vi "CompareWfm.vi"() -> ()   [LabVIEW 2022 SP3]
uses:
  <vilib>/Native 3D Graph/xcontrol/3DPC_SurfacePlot.xctl
  PreferencesControl.ctl
  <vilib>/Native 3D Graph/classes/Base Datatype.lvclass
panel:
  in  "Tab Control 2":enum32{"FRF", "Phase", "Nyquist"}(tab)
  out "Average FRF":cluster{dbl, "df":dbl, dbl[]}[](graph)
  out "Coherence":cluster{dbl, "df":dbl, dbl[]}(graph)
  in  "Remember":bool
  in  "Save":bool
  out "Phase":cluster{"t0":dbl, "dt":dbl, "Y":dbl[]}(graph)
  out "Energy":cluster{"x0":dbl, "df":dbl, dbl[]}[](graph)
  out "Nyquist Plot":cluster{dbl[], dbl[]}(graph)
  out "3D Nyquist":refnum<class "Base Datatype.lvclass">[](xcontrol)
  in  "Method":enum16{"Sqrt(H1H2)", "H1", "H2"}(ring)
  in  "sort by":enum16{"Title", "Hammer Hit"}(ring)
  in  "revert":bool
  in  "Tab Control":enum32{"Graphs", "Setttings", "Manipulation"}(tab)
  out "Mic Spectrum":cluster{dbl, "df":dbl, "FFT {X}":dbl[]}[](graph)
  out "Hammer Data":cluster{dbl, "dt":dbl, "Y":dbl[]}[](graph)
  out "Hammer Spectrum":cluster{dbl, "df":dbl, "FFT {X}":dbl[]}[](graph)
  out "Microphone Data":cluster{dbl, "dt":dbl, "Y":dbl[]}[](graph)
  in  "View":u16(ring) items=["Raw", "Volts", "Units (Pa, N, etc)"]
  in  "Settings":T1={"Name of test"="", "Date"=timestamp(0 s since 1904-01-01), "Location"="", "Template"="", "Soundcard"="", "resolution"=32, "Sampling rate"=48000, "Ch1 Gain "=25.0, "Ch2 Gain"=10.0, "Sample time (s)"=0.3, "Pre-trigger (s)"=0.01, "Hammer Threshold"=10.0, "Positions"=12, "Taps/Position"=5, "Set Names"="", "Freq resolution"=10.0, "Hammer cutoff"=0.0, "Mic cutoff"=0.0, "Double bounce "=0.0, "Hammer Cal"=10.0, "dB Offset"=0.0, "Accel Cal"=10.0, "Vibrometer Cal"=0.0, "Mic Cal"=0.0, "Output"=2, "Voltage Cal"=1.0, "Vibrometer Port"="ASRL27::INSTR", "Range"=4, "High Pass"=2, "Bandwidth"=4, "X Range"=[], "Y Range"=[], "dB Spread"=0.0, "Trigger"=0, "Ch_1"=25, "Ch_2"=25, "flip?"=FALSE, "60Hz"=FALSE, "Time offset"=0.0, "Piezo Cal"=1.0, "Default Notes"=""} {"Ch_2" min=1 step=1; "Ch_1" min=1 max=100 step=1; "Trigger" items=["Hammer (force)", "Self-tap", "Spacebar"]; "Bandwidth" items=["1 kHz"=1, "5 kHz"=5, "10 kHz"=10, "25 kHz"=25, "50 kHz"=50, "100 kHz"=100]; "High Pass" items=["Off", "13 Hz", "104 Hz"]; "Range" items=["10 mm/s"=1, "20 mm/s"=2, "50 mm/s"=5, "100 mm/s"=10, "200 mm/s"=20, "500 mm/s"=50, "1 m/s"=100, "2 m/s"=200]; "Output" items=["Accelerometer", "Speed (from acceleration)", "Microphone", "Vibrometer", "Piezo"]; "Voltage Cal" format="%#_13g"; "Ch2 Gain" format="%#_13g"; "Ch1 Gain" format="%#_13g"; "Double bounce" min=0.0; "Mic cutoff" min=0.0 format="%#_4g"; "Hammer cutoff" min=0.0 format="%#_4g"; "Freq resolution" min=0.0; "Pre-trigger (s)" format="%#_13g"; "Date" format="%<%H:%M\n%d/%m/%y>T"; "resolution" items=["16 bit"=16, "24 bit"=24, "32 bit"=32]; "Sampling rate" items=["22050 samp/s"=22050, "44100 samp/s"=44100, "48000 samp/s"=48000]}
  in  "Range":cluster{dbl, dbl}(slide)={0.0, 2.4242424242424243} scale=0.0..22000.0
  in  "Vibrometer delay (msec)":dbl(slide) scale=0.2..0.3
  in  "dB Spread":dbl=40.0
  out "Path To Raw Folder":path
  in  "Test Name":string(combo)
  in  "Instrument Name":string(combo)
  in  "Raw wfm Files":i32[](listbox)
  # "Hz"
  # "dB"
  # "dB"
  # "sec"
  # "sec"
  # "mV/Pa"
  # "mV/m/s2"
  # "mV/mm/s"
  # "V/N"
  # "sec"
  # "sec"
  # "mV/N"
  # "a.u."
  # "a.u."
  # "sec"
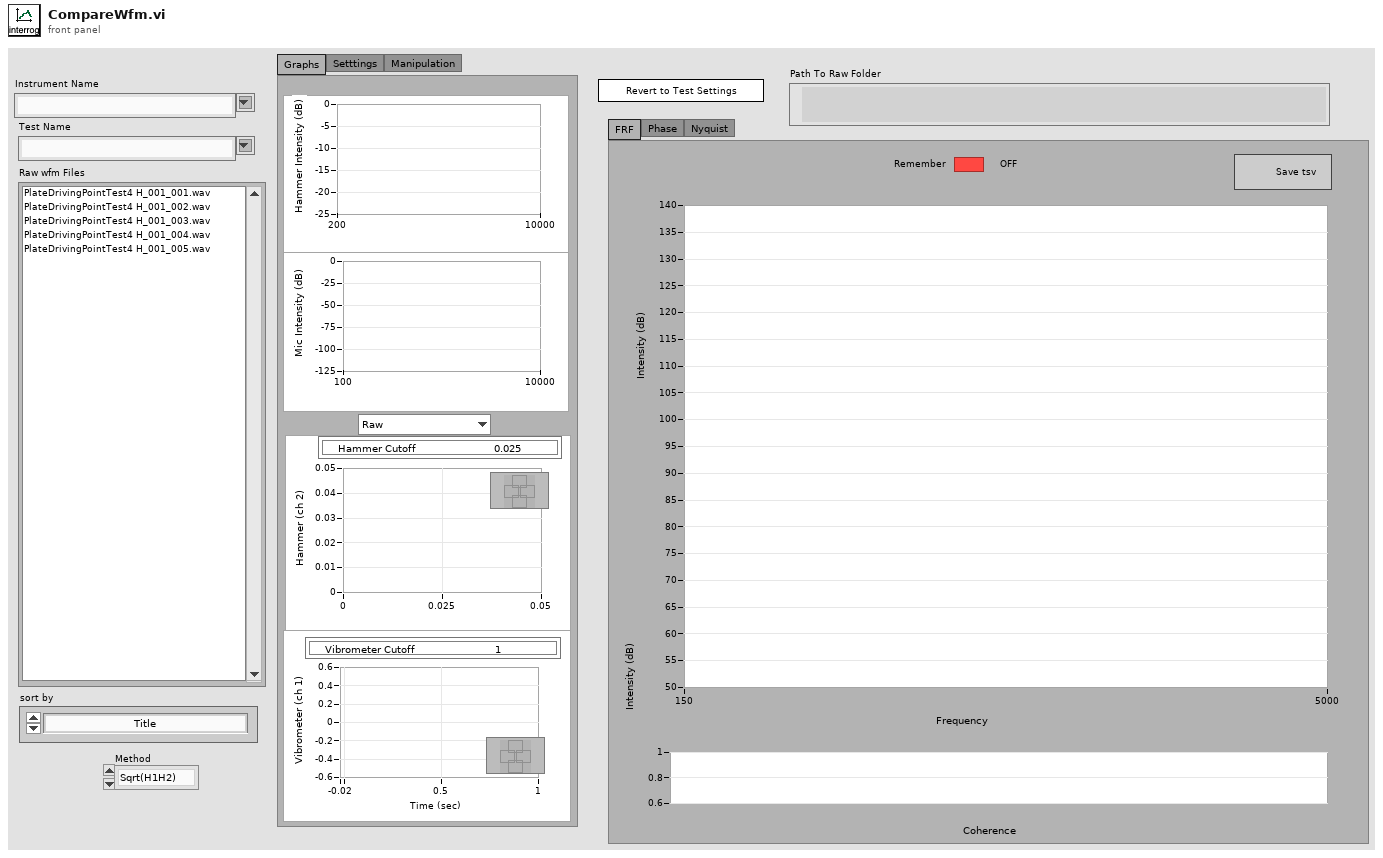
[diagram p1: front panel]
types:
  T1 = typedef "PreferencesControl.ctl" = cluster{"Name of test":string, "Date":timestamp, "Location":string, "Template":string, "Soundcard":string, "resolution":u16, "Sampling rate":u16, "Ch1 Gain ":dbl, "Ch2 Gain":dbl, "Sample time (s)":dbl, "Pre-trigger (s)":dbl, "Hammer Threshold":dbl, "Positions":i16, "Taps/Position":i16, "Set Names":string, "Freq resolution":dbl, "Hammer cutoff":dbl, "Mic cutoff":dbl, "Double bounce ":dbl, "Hammer Cal":dbl, "dB Offset":dbl, "Accel Cal":dbl, "Vibrometer Cal":dbl, "Mic Cal":dbl, "Output":u16, "Voltage Cal":dbl, "Vibrometer Port":refnum<visa-resource-name>, "Range":u16, "High Pass":u16, "Bandwidth":u16, "X Range":cluster{"Minimum":dbl, "Maximum":dbl, "Increment":dbl, "Minor Increment":dbl, "Start":dbl}[], "Y Range":cluster{"Minimum":dbl, "Maximum":dbl, "Increment":dbl, "Minor Increment":dbl, "Start":dbl}[], "dB Spread":dbl, "Trigger":u16, "Ch_1":u8, "Ch_2":u8, "flip?":bool, "60Hz":bool, "Time offset":dbl, "Piezo Cal":dbl, "Default Notes":string}
  T2 = typedef "LVRangeTypeDef.ctl" = cluster{"Minimum":dbl, "Maximum":dbl, "Increment":dbl, "Minor Increment":dbl, "Start":dbl}
  T3 = enum8{"Enabled", "Disabled", "Disabled and Grayed Out"}
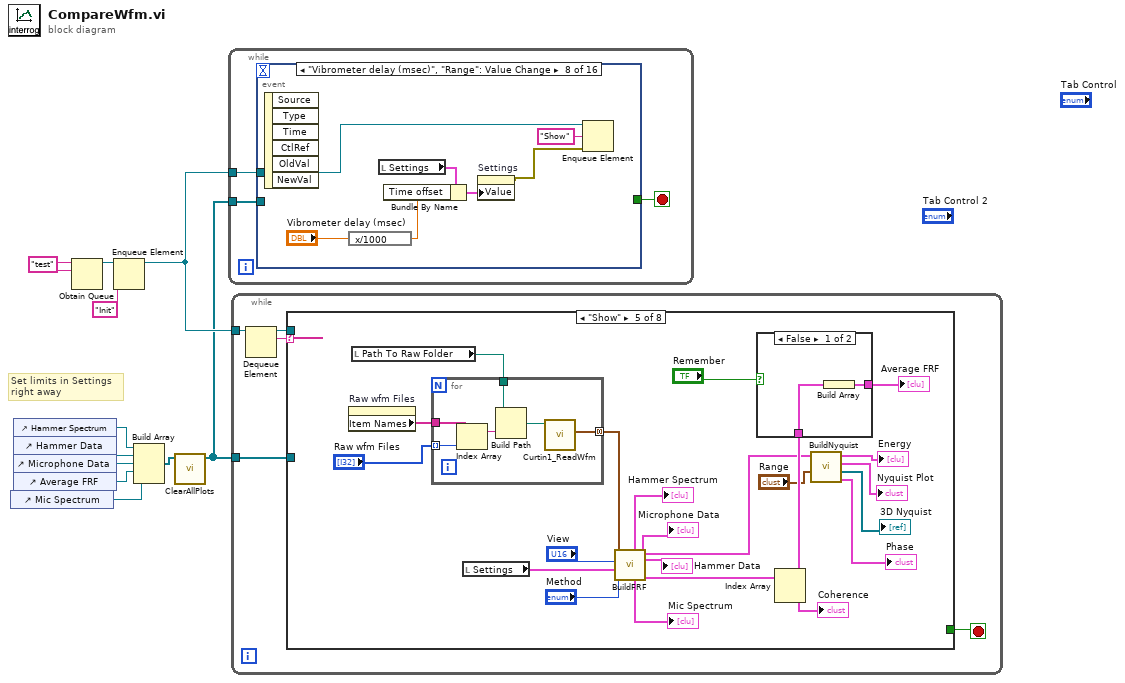
[diagram p0: block diagram]
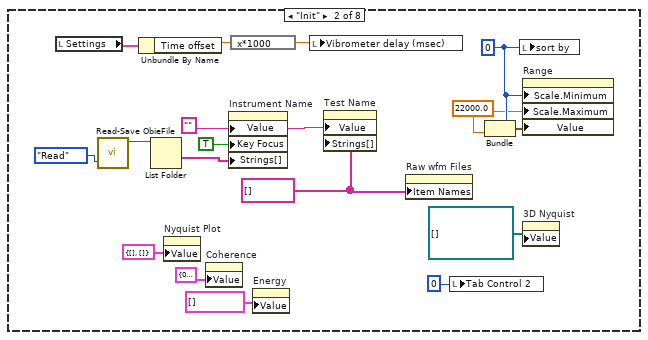
[diagram p3: hidden frame]
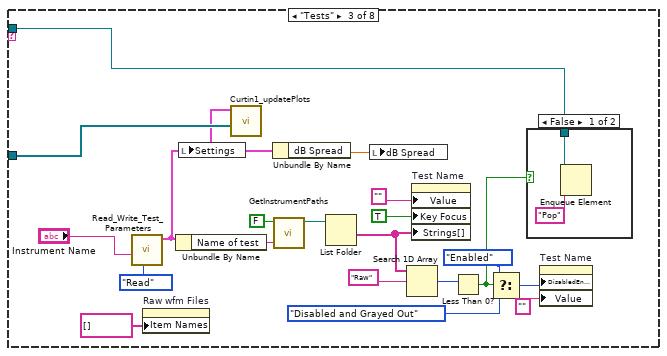
[diagram p4: hidden frame]
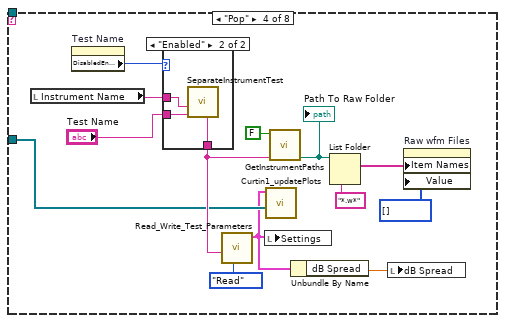
[diagram p6: hidden frame]
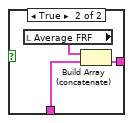
[diagram p8: hidden frame]
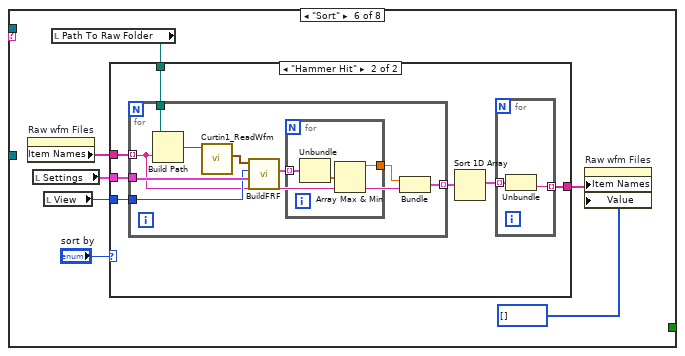
[diagram p9: hidden frame]
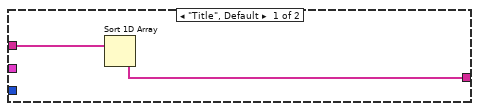
[diagram p10: hidden frame]
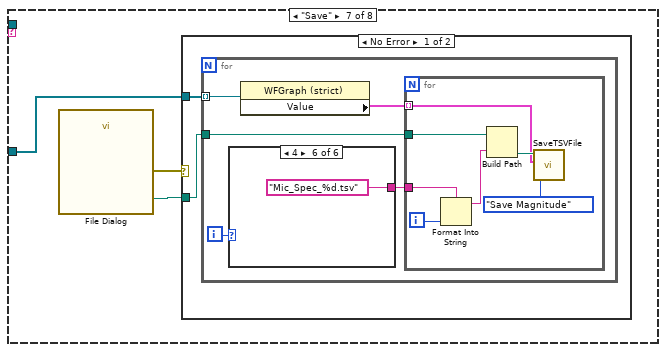
[diagram p11: hidden frame]
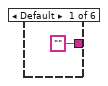
[diagram p12: hidden frame]
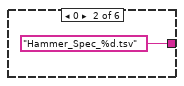
[diagram p13: hidden frame]
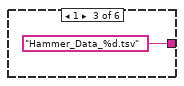
[diagram p14: hidden frame]
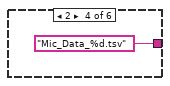
[diagram p15: hidden frame]
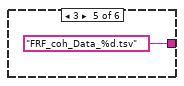
[diagram p16: hidden frame]
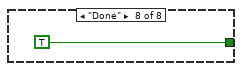
[diagram p18: hidden frame]
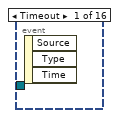
[diagram p19: hidden frame]
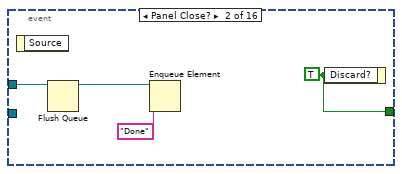
[diagram p20: hidden frame]
diagram:
  w8 = "test" ("element")
  # "Set limits in Settings \nright away"
  n1 = control-ref of="Mic Spectrum"() -> (w1:refnum<vi>)
  n2 = control-ref of="Hammer Spectrum"() -> (w3:refnum<vi>)
  n3 = control-ref of="Hammer Data"() -> (w4:refnum<vi>)
  n4 = control-ref of="Microphone Data"() -> (w5:refnum<vi>)
  n5 = control-ref of="Average FRF"() -> (w6:refnum<vi>)
  n6 = Obtain Queue(name (unnamed)=w8, element data type=w8) -> (queue out=w10:refnum<queue>)  [unwired: 3 in, 2 out]
  n7 = Enqueue Element(queue=w10, element="Init") -> (queue out=w7:refnum<queue>)  [unwired: 2 in, 2 out]
  n8 = Build Array(w3, w4, w5, w6, w1) -> (w2:refnum<vi>[])
  n9 = call "ClearAllPlots.vi"("Array"=w2) -> ()  [unwired: 11 in]
  n10 = while {
    tunnel: w7 -> [w12]
    tunnel: w2 -> [w11]
    stop <- w13 stop-if-true
    n11 = event shown="[7] \"Vibrometer delay (msec)\", \"Range\": Value Change" {
      selector: _ -> [_ _ _ _ _ _ _ _ _ _ _ _ _ _ _ _]
      dyn-events: _ -> [_ _ _ _ _ _ _ _ _ _ _ _ _ _ _ _]
      timeout: _ -> [_ _ _ _ _ _ _ _ _ _ _ _ _ _ _ _]
      tunnel: [_ w17 _ _ _ _ _ _ _ _ _ _ _ _ _ _] -> w13
      tunnel: w12 -> [_ w15 w18 w20 w22 _ _ w43 _ _ _ w59 w64 w72 w74 _]
      tunnel: w11 -> [_ _ _ _ _ _ _ _ _ _ _ _ w61 _ _ _]
      event Timeout {
        n12 = event-data() -> ()  [unwired: 1 in, 3 out]
      }
      event Panel Close? {
        w17 = TRUE ("Discard?")
        n13 = event-data() -> ()  [unwired: 1 in, 1 out]
        n14 = Flush Queue(queue=w15) -> (queue out=w14:refnum<queue>)  [unwired: 1 in, 2 out]
        n15 = Enqueue Element(queue=w14, element="Done") -> ()  [unwired: 2 in, 3 out]
        n16 = event-data("Discard?"=w17) -> ()  [unwired: 1 in, 1 out]
      }
      event "Instrument Name": Value Change {
        n17 = event-data() -> ()  [unwired: 1 in, 1 out]
        n18 = Enqueue Element(queue=w18, element="Tests") -> ()  [unwired: 2 in, 3 out]
      }
      event "Test Name": Value Change {
        n19 = event-data() -> ()  [unwired: 1 in, 1 out]
        n20 = Enqueue Element(queue=w20, element="Pop") -> ()  [unwired: 2 in, 3 out]
      }
      event "Raw wfm Files", "View": Value Change {
        n21 = event-data() -> ()  [unwired: 1 in, 1 out]
        n22 = Enqueue Element(queue=w22, element="Show") -> ()  [unwired: 2 in, 3 out]
      }
      event "Hammer Data", "Hammer Spectrum", "Microphone Data": Mouse Up {
        n23 = event-data() -> ("CtlRef"=w24:refnum<vi>, "PlatMods.Shift"=w28:bool)  [unwired: 1 in]
        n24 = property on="Raw wfm Files" class="LstBox (strict)"() -> ("Item Names"=w27:string[], "Value"=w26:i32[])  [unwired: 2 in, 2 out]
        n25 = for {
          tunnel: w27 -> [w31]
          tunnel: w26 -> [w30] mode=indexing
          tunnel: [w29] -> w25 mode=indexing
          n26 = Index Array(array=w31, index=w30) -> (element=w29:string)
        }
        n27 = case shown="True" w28 {
          tunnel: w24 -> [_ w34]
          tunnel: w25 -> [_ w32]
          frame False {
          }
          frame True {
            n28 = local read "dB Spread"() -> (w33:dbl)
            n29 = call "GraphZoom.vi"("Names"=w32, "dB Range"=w33, "Graph"=w34) -> ()  [unwired: 9 in]
          }
        }
      }
      event "Average FRF": Mouse Up {
        n30 = event-data() -> ("CtlRef"=w36:refnum<vi>, "PlatMods.Shift"=w37:bool)  [unwired: 1 in]
        n31 = case shown="True" w37 {
          tunnel: w36 -> [_ w40]
          tunnel: string[] ["Average FRF"] ("Names") -> [_ w38]
          frame False {
          }
          frame True {
            n32 = local read "dB Spread"() -> (w39:dbl)
            n33 = call "GraphZoom.vi"("Names"=w38, "dB Range"=w39, "Graph"=w40) -> ()  [unwired: 9 in]
          }
        }
      }
      event "Vibrometer delay (msec)", "Range": Value Change {
        n34 = event-data() -> ()  [unwired: 1 in, 6 out]
        n35 = expression code="x/1000"("Vibrometer delay (msec)") -> (w45:dbl)
        n36 = local read "Settings"() -> (w47:T1)
        n37 = Bundle By Name(cluster=w47, "Time offset"=w45) -> (w42:T1)
        n38 = property on="Settings" class="Clust (strict)"("Value"=w42) -> (error out=w41:errorcluster)  [unwired: 2 in, 1 out]
        n39 = Enqueue Element(queue=w43, element="Show", error in (no error)=w41) -> ()  [unwired: 1 in, 3 out]
      }
      event "Microphone Data": Cursor Move {
        n40 = event-data() -> ("CursLoc.X"=w48:dbl)  [unwired: 1 in]
        n41 = property on="Mic cutoff" class="DigNum (strict)"("Val(Sgnl)"=w48) -> ()  [unwired: 2 in, 2 out]
      }
      event "Hammer Data": Cursor Move {
        n42 = event-data() -> ("CursIdx"=w51:i32, "CursLoc.X"=w50:dbl, "CursLoc.Y"=w49:dbl)  [unwired: 1 in]
        n43 = case shown="0" w51 {
          tunnel: w50 -> [w52 _]
          tunnel: w49 -> [_ w53]
          frame 0 {
            n44 = property on="Hammer cutoff" class="DigNum (strict)"("Val(Sgnl)"=w52) -> ()  [unwired: 2 in, 2 out]
          }
          frame Default {
            n45 = property on="Hammer Threshold" class="DigNum (strict)"("Val(Sgnl)"=w53) -> ()  [unwired: 2 in, 2 out]
          }
        }
      }
      event "Average FRF": Scale Range Change {
        n46 = event-data() -> ("Kind"=w54:enum16{"X-Scale", "Y-Scale", "Z-Scale"}, "NewRange"=w55:T2)  [unwired: 1 in]
        n47 = case shown="\"X-Scale\"" w54 {
          tunnel: w55 -> [_ w56]
          frame Default {
          }
          frame "X-Scale" {
            n48 = property on="Coherence" class="WFGraph (strict)"("XScale.Range"=w56) -> ()  [unwired: 2 in, 2 out]
          }
        }
      }
      event "sort by": Value Change {
        n49 = event-data() -> ()  [unwired: 1 in, 1 out]
        n50 = Enqueue Element(queue=w59, element="Sort") -> (queue out=w57:refnum<queue>)  [unwired: 2 in, 2 out]
        n51 = Enqueue Element(queue=w57, element="Show") -> ()  [unwired: 2 in, 3 out]
      }
      event Value Change {
        n52 = event-data() -> ("NewVal"=w62:T1)  [unwired: 1 in]
        n53 = flat-sequence {
          tunnel: w64 -> [w67]
          tunnel: [w67] -> w63
          tunnel: w62 -> [w66]
          tunnel: w61 -> [w65]
          tunnel: w63 -> [w70]
          frame #0 {
            n54 = disable-structure shown="Disabled" {
              disable-tunnel: w66 -> [w69 _]
              disable-tunnel: w65 -> [w68 _]
              frame Disabled {
                n55 = call "Curtin1_updatePlots.vi"("plots"=w68, "Settings"=w69) -> ()  [unwired: 10 in]
              }
              frame Enabled {
              }
            }
          }
          frame #1 {
            n56 = Enqueue Element(queue=w70, element="Show") -> ()  [unwired: 2 in, 3 out]
          }
        }
      }
      event "Method": Value Change {
        n57 = event-data() -> ()  [unwired: 1 in, 5 out]
        n58 = Enqueue Element(queue=w72, element="Show") -> ()  [unwired: 2 in, 3 out]
      }
      event "Save": Value Change {
        n59 = event-data() -> ()  [unwired: 1 in, 1 out]
        n60 = Enqueue Element(queue=w74, element="Save") -> ()  [unwired: 2 in, 3 out]
      }
      event "revert": Value Change {
        n61 = event-data() -> ()  [unwired: 1 in, 1 out]
        n62 = local read "Instrument Name"() -> (w79:string)
        n63 = call "Read_Write_Test_Parameters.vi"("Task"=enum16{"Save", "Read", "Clear"}."Read", "Instrument Name"=w79) -> ("Exists?"=w78:bool, "Settings"=w76:T1)  [unwired: 8 in]
        n64 = case shown="True" w78 {
          tunnel: w76 -> [_ w80]
          frame False {
          }
          frame True {
            n65 = property on="Settings" class="Clust (strict)"("Val(Sgnl)"=w80) -> ()  [unwired: 2 in, 2 out]
          }
        }
      }
    }
  }
  n66 = while {
    tunnel: w7 -> [w85]
    tunnel: w2 -> [w82]
    stop <- w83 stop-if-true
    n67 = Dequeue Element(queue=w85) -> (queue out=w81:refnum<queue>, element=w84:string)  [unwired: 2 in, 2 out]
    n68 = case shown="\"Show\"" w84 {
      tunnel: [_ _ _ _ _ _ _ TRUE ("Discard?")] -> w83
      tunnel: w82 -> [_ _ w116 w128 _ _ w205 _]
      tunnel: w81 -> [_ _ w104 _ _ _ _ _]
      frame Default {
      }
      frame "Init" {
        w88 = 22000.0 ("Scale.Range:Maximum")
        w89 = 0
        w97 = string[] [] ("Strings []")
        w98 = ""
        n69 = local read "Settings"() -> (w95:T1)
        n70 = call "Read-Save ObieFile.vi"("Task"=enum16{"Save", "Read"}."Read") -> ("DataPath Out"=w101:path)  [unwired: 8 in, 2 out]
        n71 = Unbundle By Name(w95) -> ("Time offset"=w94:dbl)
        n72 = List Folder(path=w101) -> (folder names=w102:string[])  [unwired: 3 in, 3 out]
        n73 = property on="Nyquist Plot" class="XYGraph (strict)"("Value"=cluster{dbl[], dbl[]} {[], []} ("Nyquist Plot")) -> ()  [unwired: 2 in, 2 out]
        n74 = property on="Coherence" class="WFGraph (strict)"("Value"=cluster{dbl, "df":dbl, dbl[]} {0.0, "df"=0.0, []}) -> ()  [unwired: 2 in, 2 out]
        n75 = property on="Instrument Name" class="CmbBox"("Value"=w98, "Key Focus"=TRUE, "Strings[]"=w102) -> ()  [unwired: 2 in, 2 out]
        n76 = expression code="x*1000"(w94) -> (w86:dbl)
        n77 = property on="Energy" class="WFGraph (strict)"("Value"=cluster{"x0":dbl, "df":dbl, dbl[]}[] [] ("Energy")) -> ()  [unwired: 2 in, 2 out]
        n78 = local write "Vibrometer delay (msec)"(w86) -> ()
        n79 = property on="Test Name" class="CmbBox"("Value"=w98, "Strings[]"=w97) -> ()  [unwired: 2 in, 2 out]
        n80 = property on="Raw wfm Files" class="LstBox (strict)"("Item Names"=w97) -> ()  [unwired: 2 in, 2 out]
        n81 = local write "Tab Control 2"(0) -> ()
        n82 = Bundle(w89, "Scale.Range:Maximum"=w88) -> (w87:cluster{i32, "Scale.Range:Maximum":dbl})  [unwired: 1 in]
        n83 = local write "sort by"(w89) -> ()
        n84 = property on="Range" class="Slide (strict)"("Scale.Minimum"=w89, "Scale.Maximum"=w88, "Value"=w87) -> ()  [unwired: 2 in, 2 out]
        n85 = property on="3D Nyquist" class="LabVIEW 3D Graph (strict)"("Value"=refnum<class "Base Datatype.lvclass">[] [] ("3D Nyquist")) -> ()  [unwired: 2 in, 2 out]
      }
      frame "Tests" {
        n86 = call "Read_Write_Test_Parameters.vi"("Task"=enum16{"Save", "Read", "Clear"}."Read", "Instrument Name"="Instrument Name") -> ("Settings"=w114:T1)  [unwired: 8 in, 1 out]
        n87 = property on="Raw wfm Files" class="LstBox (strict)"("Item Names"=string[] []) -> ()  [unwired: 2 in, 2 out]
        n88 = Unbundle By Name(w114) -> ("Name of test"=w122:string)
        n89 = local write "Settings"(w114) -> ()
        n90 = call "Curtin1_updatePlots.vi"("plots"=w116, "Settings"=w114) -> ()  [unwired: 10 in]
        n91 = Unbundle By Name(w114) -> ("dB Spread"=w117:dbl)
        n92 = call "GetInstrumentPaths.vi"("Instrument"=w122, "Build?"=FALSE) -> ("Path To Instrument Folder"=w118:path)  [unwired: 5 in, 4 out]
        n93 = List Folder(path=w118) -> (folder names=w112:string[])  [unwired: 3 in, 3 out]
        n94 = local write "dB Spread"(w117) -> ()
        n95 = Search 1D Array(1D array=w112, element="Raw") -> (index of element=w110:i32)  [unwired: 1 in]
        n96 = property on="Test Name" class="CmbBox"("Value"="", "Key Focus"=TRUE, "Strings[]"=w112) -> ()  [unwired: 2 in, 2 out]
        n97 = Less Than 0?(x=w110) -> (x < 0?=w103:bool)
        n98 = Select(t=T3."Enabled" ("Disabled"), s=w103, f=T3."Disabled and Grayed Out" ("Disabled")) -> (s? t:f=w108:T3)
        n99 = case shown="False" w103 {
          tunnel: w104 -> [w123 _]
          frame False {
            n100 = Enqueue Element(queue=w123, element="Pop") -> ()  [unwired: 2 in, 3 out]
          }
          frame True {
          }
        }
        n101 = property on="Test Name" class="CmbBox"("DisabledEnum"=w108, "Value"="") -> ()  [unwired: 2 in, 2 out]
      }
      frame "Pop" {
        n102 = local read "Instrument Name"() -> (w135:string)
        n103 = property on="Test Name" class="CmbBox"() -> ("DisabledEnum"=w125:T3)  [unwired: 2 in, 2 out]
        n104 = case shown="\"Enabled\"" w125 {
          tunnel: w135 -> [w138 w141]
          tunnel: "Test Name" -> [_ w140]
          tunnel: [w138 w139] -> w129
          frame Default {
          }
          frame "Enabled" {
            n105 = call "SeparateInstrumentTest.vi"("test in"=w140, "Instrument in"=w141) -> ("Instrument -- test out"=w139:string)  [unwired: 5 in, 4 out]
          }
        }
        n106 = call "Read_Write_Test_Parameters.vi"("Task"=enum16{"Save", "Read", "Clear"}."Read", "Instrument Name"=w129) -> ("Settings"=w126:T1)  [unwired: 8 in, 1 out]
        n107 = local write "Settings"(w126) -> ()
        n108 = call "Curtin1_updatePlots.vi"("plots"=w128, "Settings"=w126) -> ()  [unwired: 10 in]
        n109 = call "GetInstrumentPaths.vi"("Instrument"=w129, "Build?"=FALSE) -> ("Path To Raw Folder"=w137:path)  [unwired: 5 in, 4 out]
        "Path To Raw Folder" <- w137
        n110 = Unbundle By Name(w126) -> ("dB Spread"=w127:dbl)
        n111 = List Folder(path=w137, pattern="*.w*") -> (filenames=w136:string[])  [unwired: 2 in, 3 out]
        n112 = local write "dB Spread"(w127) -> ()
        n113 = property on="Raw wfm Files" class="LstBox (strict)"("Item Names"=w136, "Value"=i32[] [] ("Files")) -> ()  [unwired: 2 in, 2 out]
      }
      frame "Show" {
        n114 = property on="Raw wfm Files" class="LstBox (strict)"() -> ("Item Names"=w163:string[])  [unwired: 2 in, 2 out]
        n115 = local read "Path To Raw Folder"() -> (w161:path)
        n116 = for {
          tunnel: w163 -> [w174]
          tunnel: "Raw wfm Files" -> [w173] mode=indexing
          tunnel: w161 -> [w172]
          tunnel: [w170] -> w159 mode=concatenating
          n117 = Index Array(array=w174, index=w173) -> (element=w169:string)
          n118 = Build Path(base path=w172, name or relative path=w169) -> (appended path=w171:path)
          n119 = call "Curtin1_ReadWfm.vi"("appended path"=w171) -> ("all waveforms in record"=w170:waveform(dbl)[])  [unwired: 9 in, 1 out]
        }
        n120 = local read "Settings"() -> (w155:T1)
        n121 = call "BuildFRF.vi"("Method"="Method", "Settings"=w155, "View"="View", "Data In"=w159) -> ("Average FRF"=w153:cluster{dbl, "df":dbl, dbl[]}[], "Microphone"=→"Microphone Data":cluster{dbl, "dt":dbl, "Y":dbl[]}[], "Hammer"=→"Hammer Data":cluster{dbl, "dt":dbl, "Y":dbl[]}[], "Complex FRF"=w146:cluster{"t0":dbl, "dt":dbl, "Y":cdb[]}, "Microphone Spectra"=→"Mic Spectrum":cluster{"x0":dbl, "df":dbl, dbl[]}[], "Hammer Spectra"=→"Hammer Spectrum":cluster{dbl, "df":dbl, "FFT {X}":dbl[]}[])  [unwired: 2 in]
        n122 = Index Array(array=w153) -> (element #1=w151:cluster{dbl, "df":dbl, dbl[]}, element #2=→"Coherence":cluster{dbl, "df":dbl, dbl[]})  [unwired: 2 in]
        n123 = case shown="False" "Remember" {
          tunnel: [w165 w166] -> w152
          tunnel: w151 -> [w164 w167]
          frame False {
            n124 = Build Array(w164) -> (w165:cluster{dbl, "df":dbl, dbl[]}[])
          }
          frame True {
            n125 = local read "Average FRF"() -> (w168:cluster{dbl, "df":dbl, dbl[]}[])
            n126 = Build Array (concatenate)(w168, w167) -> (w166:cluster{dbl, "df":dbl, dbl[]}[])
          }
        }
        "Average FRF" <- w152
        n127 = call "BuildNyquist.vi"("subset"="Range", "Complex FRF"=w146) -> ("Phase"=→"Phase":cluster{"t0":dbl, "dt":dbl, "Y":dbl[]}, "plots out"=→"3D Nyquist":refnum<class "Base Datatype.lvclass">[], "Nyquist Plot"=→"Nyquist Plot":cluster{dbl[], dbl[]}, "Energy"=→"Energy":cluster{"x0":dbl, "df":dbl, dbl[]}[])  [unwired: 6 in]
      }
      frame "Sort" {
        n128 = property on="Raw wfm Files" class="LstBox (strict)"() -> ("Item Names"=w180:string[])  [unwired: 2 in, 2 out]
        n129 = local read "Settings"() -> (w179:T1)
        n130 = local read "View"() -> (w178:u16)
        n131 = local read "Path To Raw Folder"() -> (w181:path)
        n132 = case shown="\"Hammer Hit\"" "sort by" {
          tunnel: w181 -> [_ w190]
          tunnel: w180 -> [w183 w189]
          tunnel: w179 -> [_ w188]
          tunnel: w178 -> [_ w187]
          tunnel: [w182 w184] -> w177
          frame "Title", Default {
            n133 = Sort 1D Array(array=w183) -> (sorted array=w182:string[])
          }
          frame "Hammer Hit" {
            n134 = for {
              tunnel: w189 -> [w194] mode=indexing
              tunnel: w190 -> [w201]
              tunnel: w188 -> [w199]
              tunnel: w187 -> [w196]
              tunnel: [w193] -> w186 mode=indexing
              n135 = Build Path(base path=w201, name or relative path=w194) -> (appended path=w200:path)
              n136 = call "Curtin1_ReadWfm.vi"("appended path"=w200) -> ("all waveforms in record"=w198:waveform(dbl)[])  [unwired: 9 in, 1 out]
              n137 = call "BuildFRF.vi"("Settings"=w199, "View"=w196, "Data In"=w198) -> ("Hammer"=w197:cluster{dbl, "dt":dbl, "Y":dbl[]}[])  [unwired: 3 in, 5 out]
              n138 = for {
                tunnel: [w203] -> w195
                tunnel: w197 -> [w202] mode=indexing
                n139 = Unbundle(w202) -> ("Y"=w204:dbl[])  [unwired: 2 out]
                n140 = Array Max & Min(array=w204) -> (max value=w203:dbl)  [unwired: 3 out]
              }
              n141 = Bundle(w195, w194) -> (w193:cluster{dbl, string})  [unwired: 1 in]
            }
            n142 = Sort 1D Array(array=w186) -> (sorted array=w185:cluster{dbl, string}[])
            n143 = for {
              tunnel: w185 -> [w192] mode=indexing
              tunnel: [w191] -> w184 mode=indexing
              n144 = Unbundle(w192) -> (w191:string)  [unwired: 1 out]
            }
          }
        }
        n145 = property on="Raw wfm Files" class="LstBox (strict)"("Item Names"=w177, "Value"=i32[] [] ("Files")) -> ()  [unwired: 2 in, 2 out]
      }
      frame "Save" {
        n146 = call "File Dialog"() -> ("selected path"=w206:path, "error out"=w207:errorcluster)  [unwired: 12 in, 2 out]
        n147 = case shown="No Error" w207 {
          tunnel: w206 -> [w208 _]
          tunnel: w205 -> [w209 _]
          frame No Error {
            n148 = for {
              tunnel: w208 -> [w214]
              tunnel: w209 -> [w213] mode=indexing
              i -> [w211]
              n149 = case shown="4" w211 {
                tunnel: ["" ("string") "Hammer_Spec_%d.tsv" ("string") "Hammer_Data_%d.tsv" ("string") "Mic_Data_%d.tsv" ("string") "FRF_coh_Data_%d.tsv" ("string") "Mic_Spec_%d.tsv" ("string")] -> w210
                frame Default {
                }
                frame 0 {
                }
                frame 1 {
                }
                frame 2 {
                }
                frame 3 {
                }
                frame 4 {
                }
              }
              n150 = property class="WFGraph (strict)"(reference=w213) -> ("Value"=w212:cluster{dbl, "df":dbl, "FFT {X}":dbl[]}[])  [unwired: 1 in, 2 out]
              n151 = for {
                tunnel: w214 -> [w225]
                tunnel: w212 -> [w224] mode=indexing
                tunnel: w210 -> [w222]
                i -> [w223]
                n152 = Format Into String(format string=w222, w223) -> (resulting string=w221:string)  [unwired: 2 in, 1 out]
                n153 = Build Path(base path=w225, name or relative path=w221) -> (appended path=w226:path)
                n154 = call "SaveTSVFile.vi"("Task"=enum16{"Save Magnitude", "Save Complex"}."Save Magnitude", "FRF"=w224, "Path"=w226) -> ()  [unwired: 8 in, 1 out]
              }
            }
          }
          frame Error {
          }
        }
      }
      frame "Done" {
      }
    }
  }
